vi "Target LRN Update.vi"(7 "Learning Gains":T1, 11 "Error Lookup Table":dbl[](array[numeric])) -> (3 "Updated Feedforward Lookup Table":dbl[](array[numeric]))   [LabVIEW 2018, in "COBRA Iterative Learning Control Library.lvlib"]
uses:
  Target Learning Gains.ctl
  COBRA Iterative Learning Control Library.lvlib
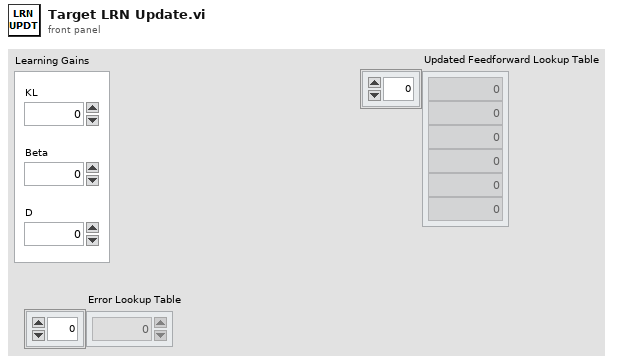
[diagram p1: front panel]
types:
  T1 = typedef "COBRA Iterative Learning Control Library.lvlib/Target Learning Gains.ctl" = cluster{"KL":dbl, "Beta":dbl, "D":i32}
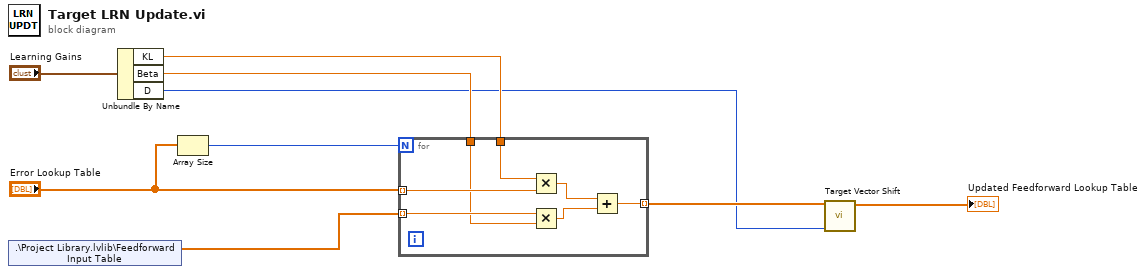
[diagram p0: block diagram]
diagram:
  n1 = shared-variable ".\\Project Library.lvlib\\Feedforward Input Table"() -> (w1:dbl[])  [unwired: 1 in, 1 out]
  n2 = Unbundle By Name("Learning Gains") -> ("KL"=w6:dbl, "Beta"=w5:dbl, "D"=w4:i32)
  n3 = Array Size(array="Error Lookup Table") -> (size(s)=w3:i32)
  n4 = for {
    N: w3 -> [_]
    tunnel: "Error Lookup Table" -> [w16] mode=indexing
    tunnel: w1 -> [w12] mode=indexing
    tunnel: [w14] -> w9 mode=indexing
    tunnel: w6 -> [w11]
    tunnel: w5 -> [w10]
    n5 = Multiply(x=w11, y=w16) -> (x*y=w15:dbl)
    n6 = Multiply(x=w12, y=w10) -> (x*y=w13:dbl)
    n7 = Add(x=w15, y=w13) -> (x+y=w14:dbl)
  }
  n8 = call "Target Vector Shift.vi"("Shift"=w4, "Input Vector"=w9) -> ("Output Vector"=→"Updated Feedforward Lookup Table":dbl[])  [unwired: 9 in]
